vi "Generate Simulated Data.vi"(7 "error in (no error)":errorcluster, 10 "Config In":T1) -> (0 "error out":errorcluster, 2 "Image Out":T6, 3 "Config Out":T1)   [LabVIEW 2019, in "Acquisition.lvlib"]
doc: "Generates sample waveforms according to the signal type in the HW Config input."
uses:
  Acquisition.lvlib
  <vilib>/vision/Image Controls.llb/IMAQ Image.ctl
  Settings/Settings.ctl
  HardwareAdapter/Support/Hardware Configuration.ctl
  Signal Type.ctl
  Logging/Logging Configuration.ctl
  HardwareAdapter/Support/Camera Configuration.ctl
  E:/DevHardSoftware/MMicroscopy/HardwareAdapter/Camera/Dependencies/PVCamNET.dll
  HardwareAdapter/Camera/Dependencies/PVCamNET.dll
  Logging/Logging.lvlib
  Settings/Settings.lvlib
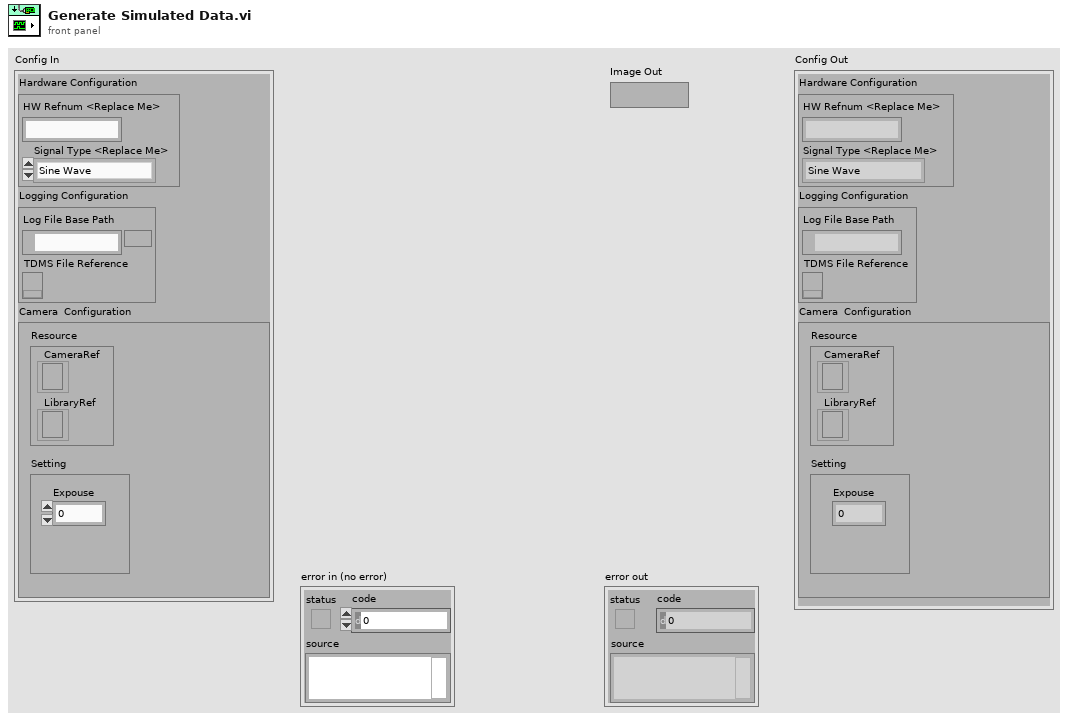
[diagram p1: front panel]
types:
  T1 = typedef "Settings.lvlib/Settings.ctl" = cluster{"Hardware Configuration":T2, "Logging Configuration":T4, "Camera Configuration":T5}
  T2 = typedef "Hardware Configuration.ctl" = cluster{"HW Refnum <Replace Me>":string, "Signal Type <Replace Me>":T3}
  T3 = typedef "Acquisition.lvlib/Signal Type.ctl" = enum16{"Sine Wave", "Square with Noise"}
  T4 = typedef "Logging.lvlib/Logging Configuration.ctl" = cluster{"Log File Base Path":path, "TDMS File Reference":refnum<k34>}
  T5 = typedef "Camera Configuration.ctl" = cluster{"Resource":cluster{"CameraRef":refnum<k24>, "LibraryRef":refnum<k24>}, "Setting":cluster{"Expouse":dbl}}
  T6 = typedef "IMAQ Image.ctl" = refnum<image>
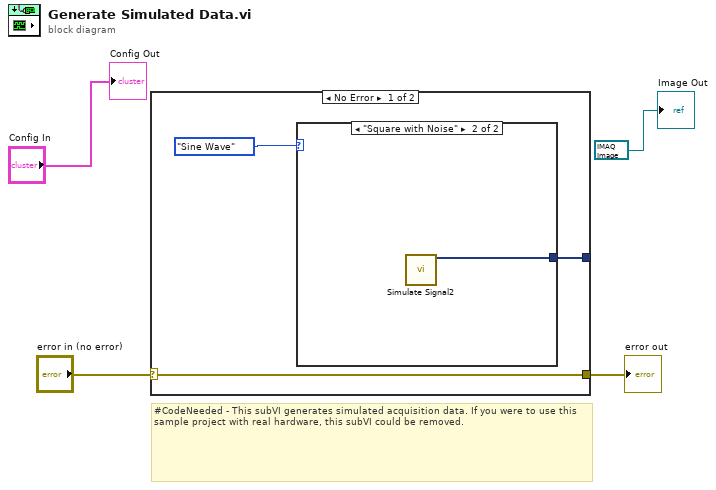
[diagram p0: block diagram]
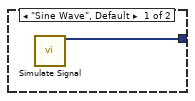
[diagram p2: hidden frame]
diagram:
  # "#CodeNeeded - This subVI generates simulated acquisition data. If you were to use this sample project with real hardware, this subVI could be removed."
  n1 = case shown="No Error" "error in (no error)" {
    selector: "error in (no error)" -> [w7 w10]
    tunnel: [w7 w10] -> w3
    tunnel: [w6 _] -> _
    frame No Error {
      n2 = case shown="\"Square with Noise\"" Signal_Type."Sine Wave" ("Signal Type") {
        tunnel: [w8 w9] -> w6
        frame "Sine Wave", Default {
          n3 = call "Simulate Signal"() -> ("Sine"=w8:dynamicdata)  [unwired: 14 in, 1 out]
        }
        frame "Square with Noise" {
          n4 = call "Simulate Signal2"() -> ("Square with Gaussian Noise"=w9:dynamicdata)  [unwired: 14 in, 1 out]
        }
      }
    }
    frame Error {
    }
  }
  "error out" <- w3
  "Image Out" <- T6 refnum ("Image Out")
  "Config Out" <- "Config In"
